vi "teste2.vi"(7 "Numeric":dbl) -> (2 "Boolean":bool)   [LabVIEW 2023]
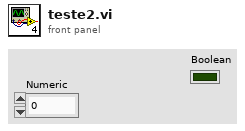
[diagram p1: front panel]
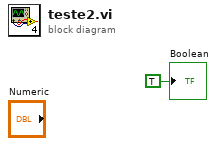
[diagram p0: block diagram]
diagram:
  "Boolean" <- TRUE ("Boolean")
